vi "Pre Launch Init.vi"(11 "前面板控制 in":refnum<class "前面板控制.lvclass"> caption="操作者输入") -> (0 "error out":errorcluster caption="错误输出", 3 "前面板控制 out":refnum<class "前面板控制.lvclass"> caption="操作者输出")   [LabVIEW 2015, in "前面板控制.lvlib" / "前面板控制.lvclass"]
doc: "(<B>Filename</B>: Actor Framework.lvlib:Actor.lvclass:Pre Launch Init.vi)\n\nDefines behavior that occurs after the Launch Nested Actor method is invoked but before the actor's Actor Core method begins running.\n\nBy default, this method does nothing. A descendant class may override it to define behavior."
uses:
  <vilib>/ActorFramework/Actor/Actor.lvclass
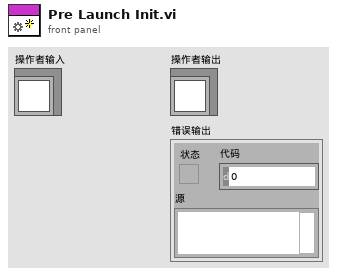
[diagram p1: front panel]
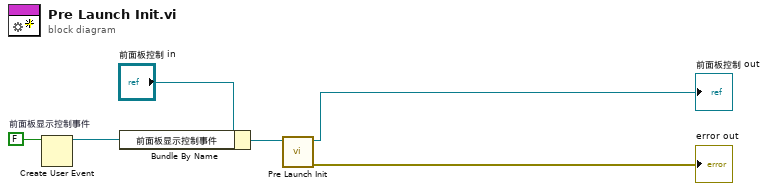
[diagram p0: block diagram]
diagram:
  w4 = FALSE  # 前面板显示控制事件
  n1 = Create User Event(user event datatype=w4) -> (user event=w1:refnum<user-event>)  [unwired: 1 in, 1 out]
  n2 = Bundle By Name(cluster="前面板控制 in", "前面板显示控制事件"=w1) -> (w2:refnum<class "前面板控制.lvclass">)
  n3 = call-parent "Pre Launch Init.vi"("Actor in"=w2) -> ("error out"=→"error out":errorcluster, "Actor out"=→"前面板控制 out":refnum<class "前面板控制.lvclass">)  [unwired: 9 in]
